vi "Constants.vi"() -> ()   [LabVIEW 2012]
uses:
  MapPOS.ctl
panel:
  out "Error Codes":errorcluster[](array[cluster])=[{"status"=TRUE, "code"=6000, "source"="Data directory no found.  App cannot start without this.\nPlease contact administrator immediatly"}, {"status"=TRUE, "code"=6001, "source"="(OmniDriver32.dll not found App cannot start without this.\nPlease contact administrator immediatly) GenerateFilePaths.vi"}, {"status"=TRUE, "code"=6002, "source"="(common32.dll not found App cannot start without this.\nPlease contact administrator immediatly) GenerateFilePaths.vi"}, {"status"=TRUE, "code"=6003, "source"="(TestConfiguration not found Loading defualt values) GenerateFilePaths.vi"}, {"status"=TRUE, "code"=6004, "source"="(EPI_Wafer_Labels.jpg not found App cannot start without this.\nPlease contact administrator immediatly) GenerateFilePaths.vi"}]
  in  "MapPOS":T1=[{"Coords"={"Horizontal"=442.6475, "Vertical"=669.9272}, "radius"=8, "state"=FALSE, "Id"="G6-E"}, {"Coords"={"Horizontal"=442.6475, "Vertical"=669.9272}, "radius"=8, "state"=FALSE, "Id"="G5-E"}, {"Coords"={"Horizontal"=364.69348, "Vertical"=668.5095}, "radius"=8, "state"=FALSE, "Id"="G4-E"}, {"Coords"={"Horizontal"=364.69348, "Vertical"=668.5095}, "radius"=8, "state"=FALSE, "Id"="G3-E"}, {"Coords"={"Horizontal"=364.69348, "Vertical"=668.5095}, "radius"=8, "state"=FALSE, "Id"="G2-E"}, {"Coords"={"Horizontal"=363.11108, "Vertical"=648.93866}, "radius"=8, "state"=FALSE, "Id"="G1-E"}, {"Coords"={"Horizontal"=447.39462, "Vertical"=126.33716}, "radius"=8, "state"=FALSE, "Id"="T6-E"}, {"Coords"={"Horizontal"=445.81226, "Vertical"=162.7318}, "radius"=8, "state"=FALSE, "Id"="T5-E"}, {"Coords"={"Horizontal"=445.81226, "Vertical"=162.7318}, "radius"=8, "state"=FALSE, "Id"="T4-E"}, {"Coords"={"Horizontal"=364.85822, "Vertical"=128.33716}, "radius"=8, "state"=FALSE, "Id"="T3-E"}, {"Coords"={"Horizontal"=364.27585, "Vertical"=145.16092}, "radius"=8, "state"=FALSE, "Id"="T2-E"}, {"Coords"={"Horizontal"=364.69348, "Vertical"=164.7318}, "radius"=8, "state"=FALSE, "Id"="T1-E"}, {"Coords"={"Horizontal"=668.6743, "Vertical"=374.1877}, "radius"=9, "state"=FALSE, "Id"="R3-E"}, {"Coords"={"Horizontal"=651.1034, "Vertical"=374.1877}, "radius"=8, "state"=FALSE, "Id"="R2-E"}, {"Coords"={"Horizontal"=630.95013, "Vertical"=372.60535}, "radius"=9, "state"=FALSE, "Id"="R1-E"}, {"Coords"={"Horizontal"=671.6743, "Vertical"=444.81226}, "radius"=8, "state"=FALSE, "Id"="R6-E"}, {"Coords"={"Horizontal"=652.6858, "Vertical"=445.977}, "radius"=8, "state"=FALSE, "Id"="R5-E"}, {"Coords"={"Horizontal"=634.1149, "Vertical"=444.81226}, "radius"=8, "state"=FALSE, "Id"="R4-E"}, {"Coords"={"Horizontal"=178.97318, "Vertical"=442.22986}, "radius"=8, "state"=FALSE, "Id"="L6-E"}, {"Coords"={"Horizontal"=160.4023, "Vertical"=442.22986}, "radius"=8, "state"=FALSE, "Id"="L5-E"}, {"Coords"={"Horizontal"=142.57854, "Vertical"=442.22986}, "radius"=8, "state"=FALSE, "Id"="L4-2"}, {"Coords"={"Horizontal"=179.97318, "Vertical"=366.11108}, "radius"=8, "state"=FALSE, "Id"="L3-E"}, {"Coords"={"Horizontal"=159.56705, "Vertical"=365.11108}, "radius"=8, "state"=FALSE, "Id"="L2-E"}, {"Coords"={"Horizontal"=142.99617, "Vertical"=364.69348}, "radius"=8, "state"=FALSE, "Id"="L1-E"}, {"Coords"={"Horizontal"=444.39462, "Vertical"=364.52872}, "radius"=9, "state"=FALSE, "Id"="D"}, {"Coords"={"Horizontal"=444.39462, "Vertical"=442.22986}, "radius"=9, "state"=FALSE, "Id"="C"}, {"Coords"={"Horizontal"=368.27585, "Vertical"=441.22986}, "radius"=9, "state"=FALSE, "Id"="B"}, {"Coords"={"Horizontal"=367.85822, "Vertical"=364.52872}, "radius"=9, "state"=FALSE, "Id"="A"}]
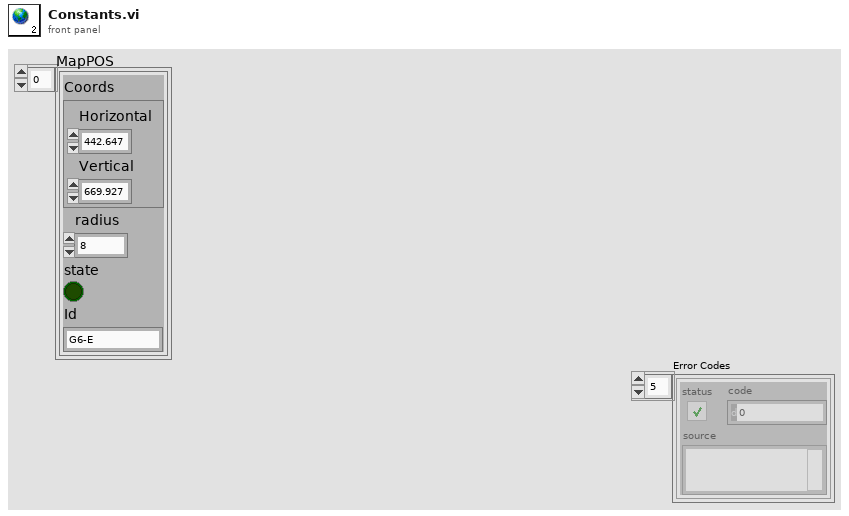
[diagram p1: front panel]
types:
  T1 = typedef "MapPOS.ctl" = cluster{"Coords":cluster{"Horizontal":sgl, "Vertical":sgl}, "radius":i32, "state":bool, "Id":string}[]
diagram:
